vi "Op-Amp Test System.vi"() -> ()   [LabVIEW 2019]
uses:
  <vilib>/VirtualBench/VirtualBench.lvlib
  <vilib>/VirtualBench/_PS Configure Voltage Output0.vi
  <vilib>/VirtualBench/_MSO Configure Digital Edge Trigger0.vi
  <vilib>/VirtualBench/_MSO Configure Analog Edge Trigger0.vi
  <vilib>/VirtualBench/_MSO Configure Digital Pattern Trigger0.vi
  <vilib>/VirtualBench/_FGEN Configure Standard Waveform4.vi
  <vilib>/VirtualBench/_MSO Configure Timing12.vi
  <vilib>/Utility/error.llb/DialogType.ctl
  <vilib>/VirtualBench/_MSO Configure Analog Channel28.vi
  <vilib>/VirtualBench/_DMM Configure Measurement2.vi
  <vilib>/VirtualBench/_FGEN Configure Standard Waveform14.vi
  <vilib>/VirtualBench/_MSO Configure Analog Channel29.vi
  <vilib>/DigilentWF/DigilentWF.lvlib
panel:
  out "测试进度":u8(slide)=100 caption="Testing..." scale=0.0..100.0
  in  "开始测试":bool caption="Start"
  out "Slew Rate(V/us)":dbl format="%#.2f"
  out "Iin+(mA)":dbl format="%#.2g"
  out "Voffset(mV)":dbl=0.00017364742031570723 format="%#.2f"
  out "Iin-(mA)":dbl format="%#.2g"
  in  "图表选项卡":enum32{"Time Domain", "Frequency Domain"}(tab)=enum."Frequency Domain"
  out "Time Domain":waveform(dbl)(graph)={"t0"=timestamp(3648703829.272387 s since 1904-01-01), "dt"=5e-06, "Y"=[], "attributes"=variant("NI_ChannelName"=variant(string "mso/1"), "NI_UnitDescription"=variant(string "Volts"))}
  out "Amplitude-frequency":cluster{dbl[], dbl[]}(graph) caption="Amplitude-frequency characteristic"
  out "PSRR(dB)":dbl format="%#.1f"
  out "KCMRR(dB)":dbl format="%#.1f"
  out "Iin_mean(mA)":dbl format="%#.2g"
  out "Iin_bias(mA)":dbl format="%#.5g"
  out "K0(dB)":dbl format="%#.1f"
  in  "测试参数选项卡":T1(tab)=enum."Slew Rate"
  in  "Current PWS":T2={"PWS Channel"="VB8012-3126A15/ps/+25V", "Voltage Level (V)"=10.0, "Current Limit (A)"=0.05} {"Voltage Level (V)" min=0.0 max=12.0}
  in  "DC Offset(V)":dbl=1.0 caption="DC Offset" format="%#_13g"
  in  "Waveform Function":enum16{"Sine", "Square", "Triangle/Ramp", "DC"}(ring)=enum."DC"
  in  "CMRR PWS 2":T3={"PWS Channel 2"="VB8012-3126A15/ps/-25V", "Voltage Level (V)"=[-9.5, -8.5], "Current Limit (A)"=0.05} {"Voltage Level (V)" min=-12.0 max=0.0}
  in  "CMRR PWS1":T4={"PWS Channel 1"="VB8012-3126A15/ps/+25V", "Voltage Level (V)"=[9.5, 10.5], "Current Limit (A)"=0.05} {"Voltage Level (V)" min=0.0 max=12.0}
  in  "PSRR PWS":T5={"PWS Channel"="VB8012-3126A15/ps/+25V", "Voltage Level (V)"=[9.5, 10.0], "Current Limit (A)"=0.05} {"Voltage Level (V)" min=0.0 max=12.0}
  in  "Slew Rate PWS":T2={"PWS Channel"="VB8012-3126A15/ps/+25V", "Voltage Level (V)"=10.0, "Current Limit (A)"=0.05} {"Voltage Level (V)" min=0.0 max=12.0}
  in  "Frequency":dbl=20000.0 format="%#_13g"
  in  "Slewrate Waveform":enum16{"Sine", "Square", "Triangle/Ramp", "DC"}(ring)=enum."Square" caption="Waveform Function"
  in  "Amplitude":dbl=3.0 format="%#_13g"
  in  "DC Offset":dbl format="%#_13g"
  in  "Channel":tag="VB8012-3126A15/mso/1"
  in  "Vertical Range":dbl=3.0 format="%#_13g"
  in  "Trigger Type":T6(tab)
  in  "Digital Trigger Source":tag="mso/d0" caption="Trigger Source (no change)"
  in  "Edge":i32(ring) caption="Trigger Slope (no change)" items=["Rising", "Falling", "Either"]
  in  "Level (V)":dbl=0.4 format="%0.2f"
  in  "Hysteresis (V)":dbl=0.17
  in  "Analog Trigger Source":tag="VB8012-3126A15/mso/1" caption="Trigger Source (no change)"
  in  "Slope":i32(ring) caption="Trigger Slope (no change)" items=["Rising", "Falling", "Either"]
  in  "Pattern Trigger Source":tag="mso/d0:7" caption="Trigger Source (no change)"
  in  "Trigger Pattern":string="1R0XX1X0" caption="Trigger Pattern (no change)"
  in  "BW PWS":T2={"PWS Channel"="VB8012-3126A15/ps/+25V", "Voltage Level (V)"=10.0, "Current Limit (A)"=0.05} {"Voltage Level (V)" min=0.0 max=12.0}
  in  "Slewrate Waveform":enum16{"Sine", "Square", "Triangle/Ramp", "DC"}(ring) caption="Waveform Function"
  in  "Amplitude":dbl=2.0 format="%#_13g"
  in  "DC Offset":dbl format="%#_13g"
  in  "Vertical Range":dbl=3.0 format="%#_13g"
  in  "Channel":tag="VB8012-3126A15/mso/1"
  in  "Trigger Type":T6(tab)
  in  "Digital Trigger Source":tag="mso/d0" caption="Trigger Source (no change)"
  in  "Edge":i32(ring) caption="Trigger Slope (no change)" items=["Rising", "Falling", "Either"]
  in  "Analog Trigger Source":tag="mso/1" caption="Trigger Source (no change)"
  in  "Slope":i32(ring) caption="Trigger Slope (no change)" items=["Rising", "Falling", "Either"]
  in  "Level (V)":dbl format="%0.2f"
  in  "Hysteresis (V)":dbl=0.17
  in  "Pattern Trigger Source":tag="mso/d0:7" caption="Trigger Source (no change)"
  in  "Trigger Pattern":string="1R0XX1X0" caption="Trigger Pattern (no change)"
  in  "测试机台选择":tag="VB8012-3126A15"
  # "基于IECUBE-3839的运放自动化测试程序"
  # "硬件配置"
  # "DUT测试参数"
  # "设备选择"
  # "DUT测试结果"
  # "电源配置"
  # "函数发生器配置"
  # "电源配置"
  # "电源配置"
  # "电源配置"
  # "函数发生器配置"
  # "逻辑分析仪配置"
  # "Triggers immediately after MSO Run VI executes."
  # "电源配置"
  # "函数发生器配置"
  # "逻辑分析仪配置"
  # "Triggers immediately after MSO Run VI executes."
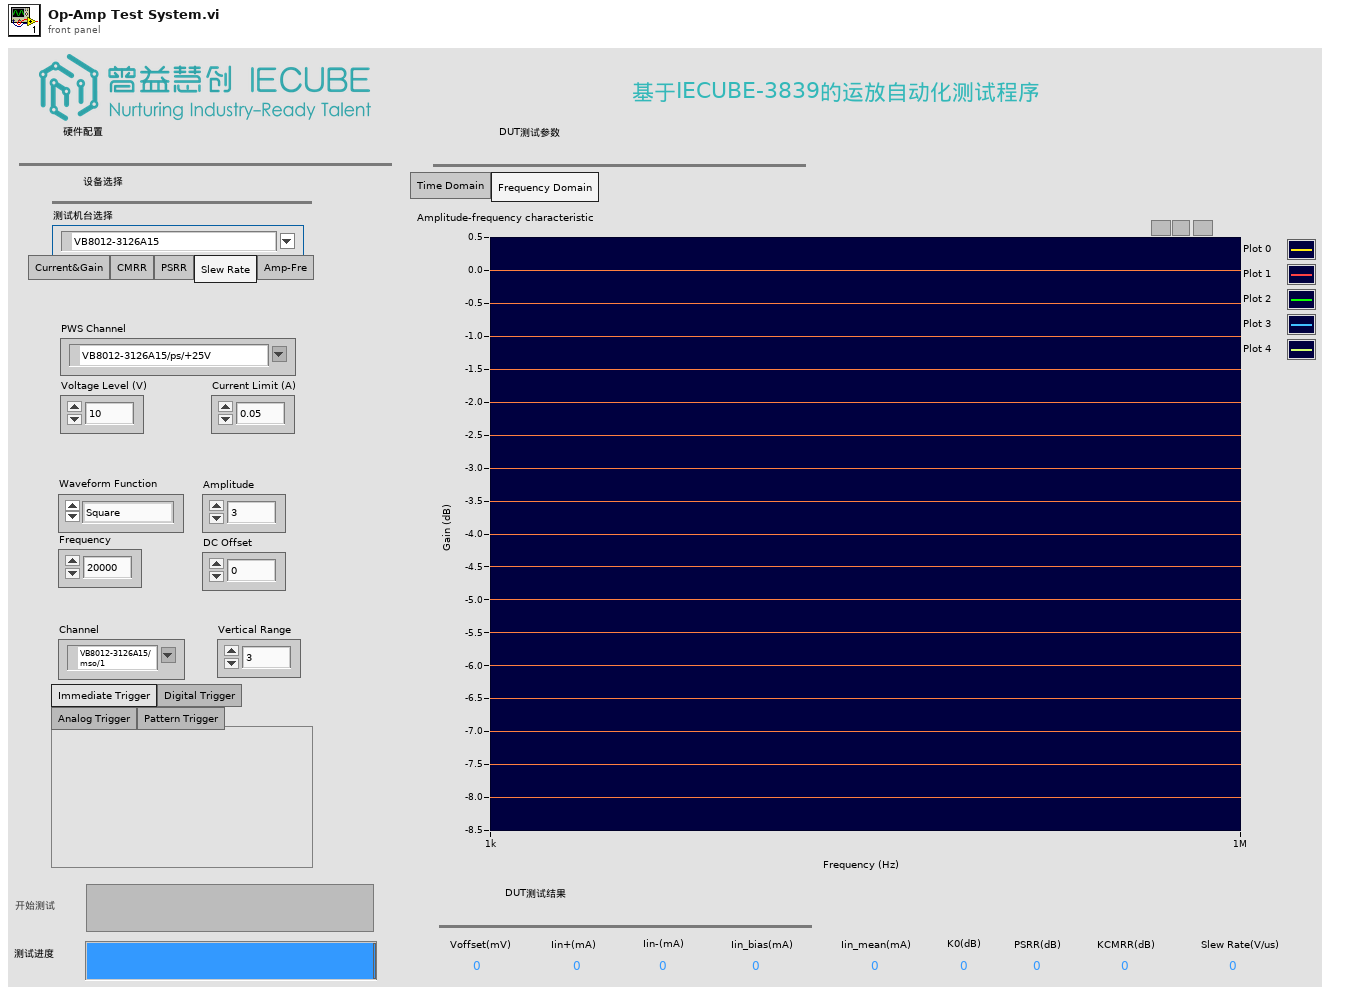
[diagram p1: front panel]
types:
  T1 = enum32{"Current&Gain", "CMRR", "PSRR", "Slew Rate", "Amp-Fre"}
  T2 = cluster{"PWS Channel":tag, "Voltage Level (V)":dbl, "Current Limit (A)":dbl}
  T3 = cluster{"PWS Channel 2":tag, "Voltage Level (V)":dbl[], "Current Limit (A)":dbl}
  T4 = cluster{"PWS Channel 1":tag, "Voltage Level (V)":dbl[], "Current Limit (A)":dbl}
  T5 = cluster{"PWS Channel":tag, "Voltage Level (V)":dbl[], "Current Limit (A)":dbl}
  T6 = enum32{"Immediate Trigger", "Digital Trigger", "Analog Trigger", "Pattern Trigger"}
  T7 = typedef "测试参数.ctl" = enum16{"Leakage Current", "Gain", "CMRR", "PSRR", "Slew Rate", "Amplitude-Frequency"}
  T8 = typedef "DialogType.ctl" = u16
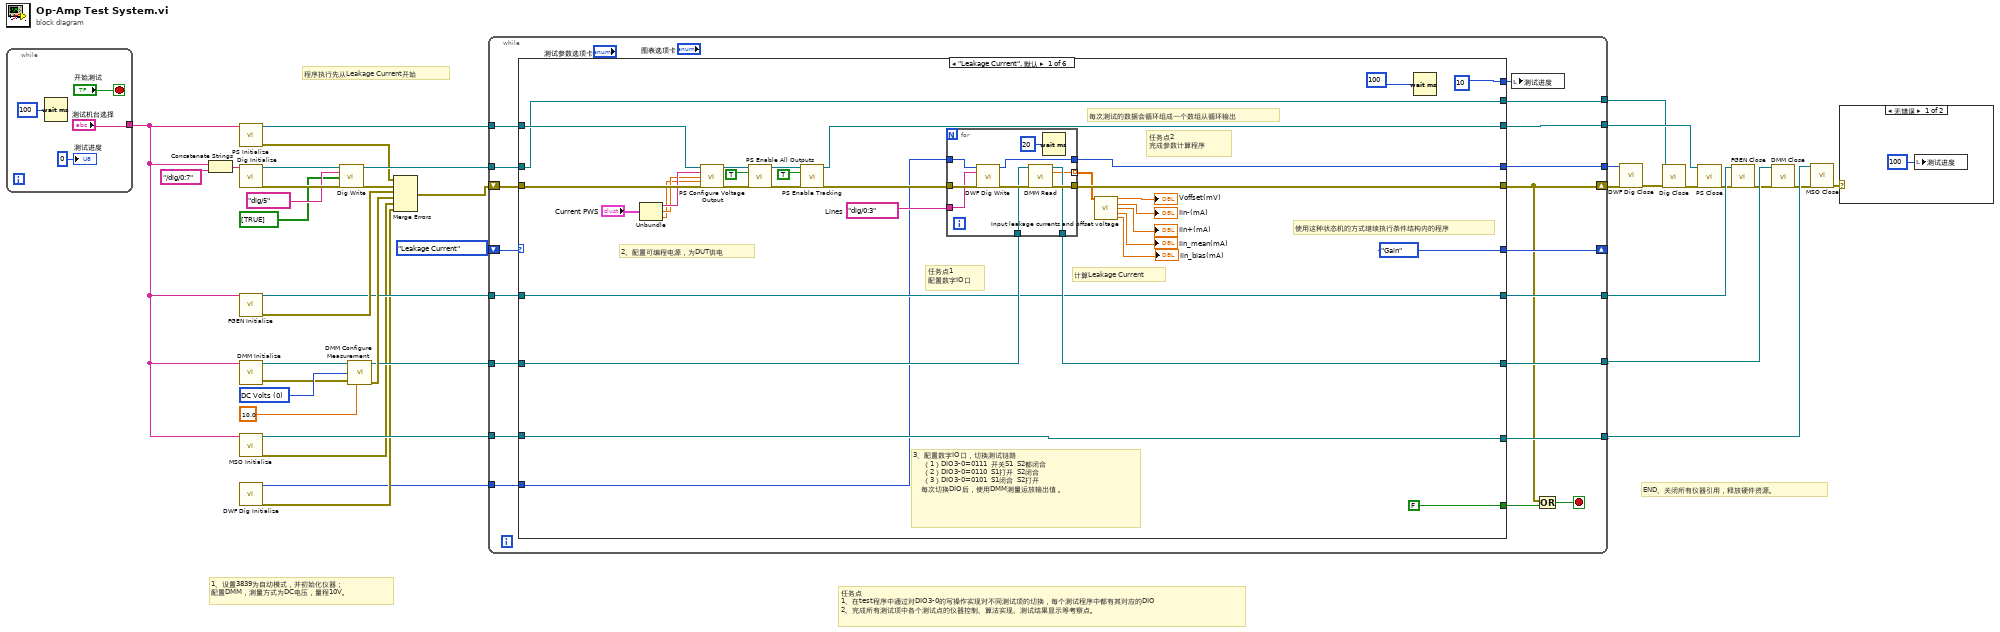
[diagram p0: block diagram]
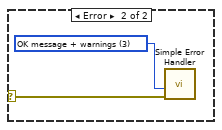
[diagram p2: hidden frame]
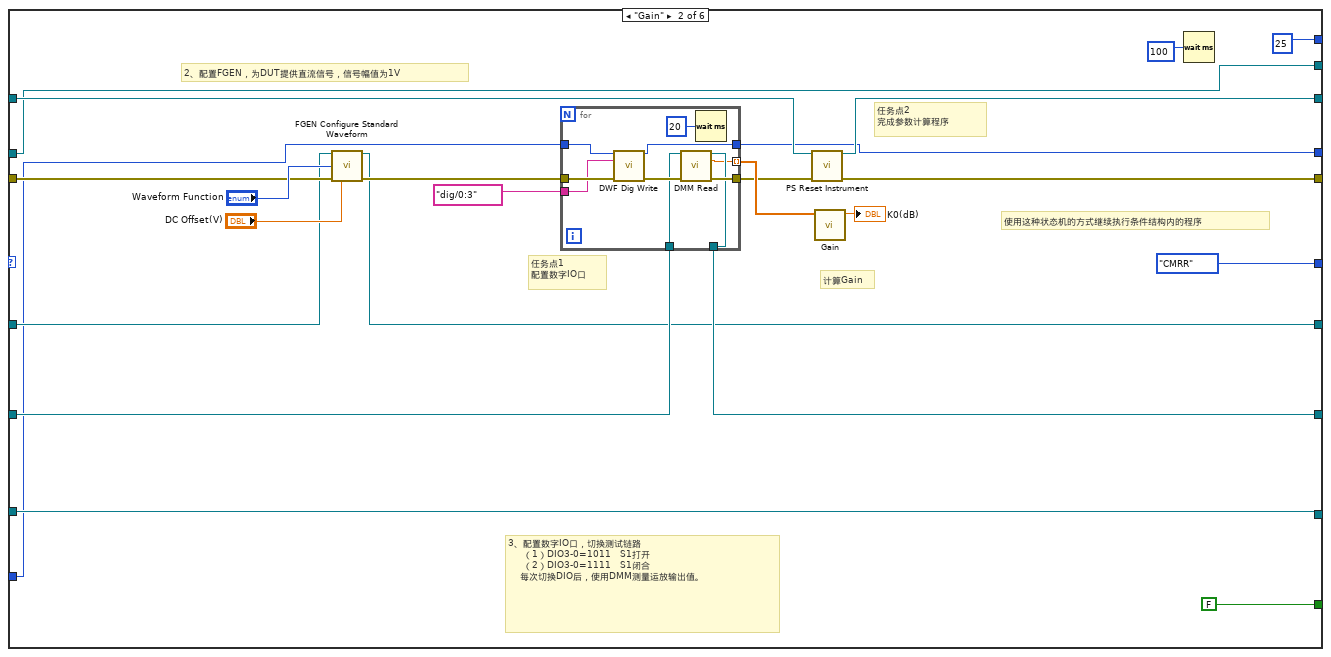
[diagram p3: hidden frame]
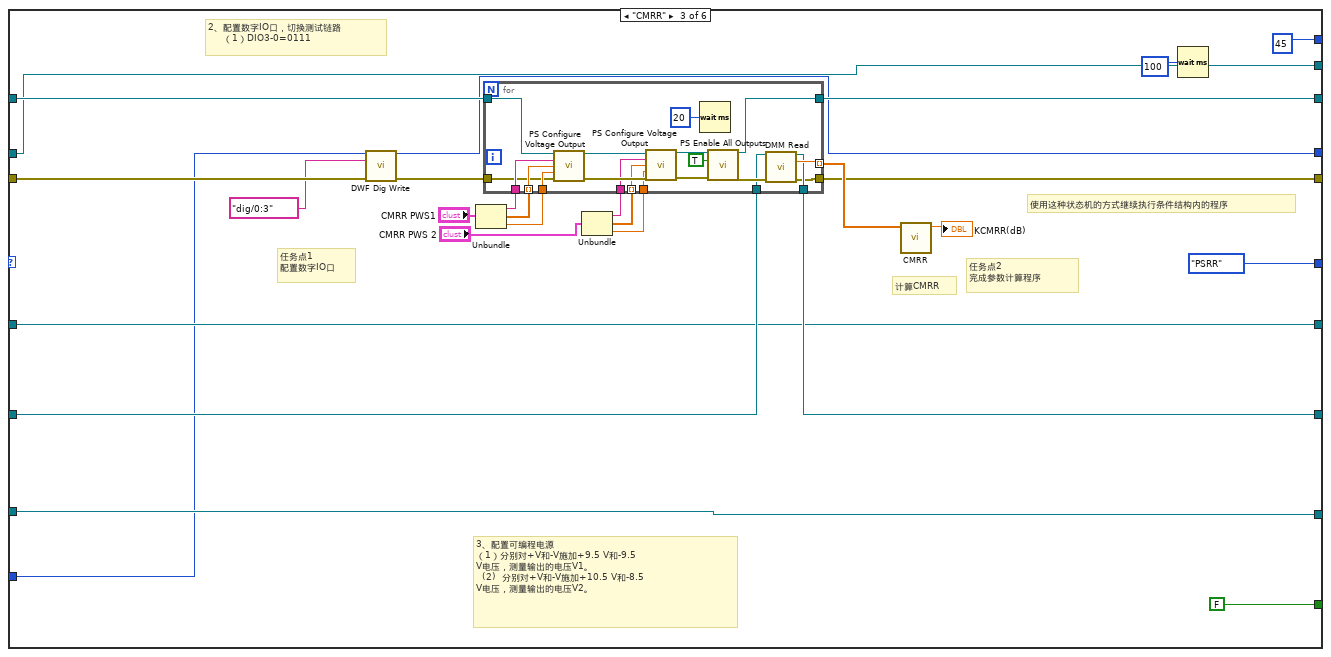
[diagram p4: hidden frame]
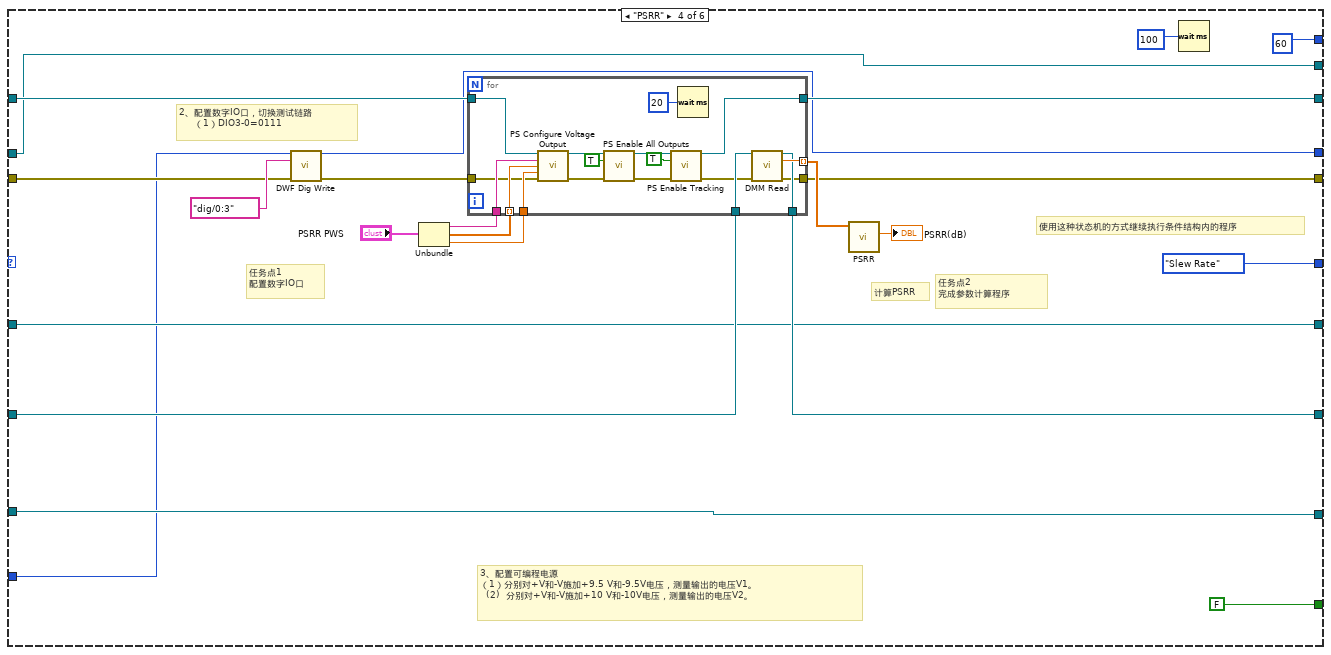
[diagram p5: hidden frame]
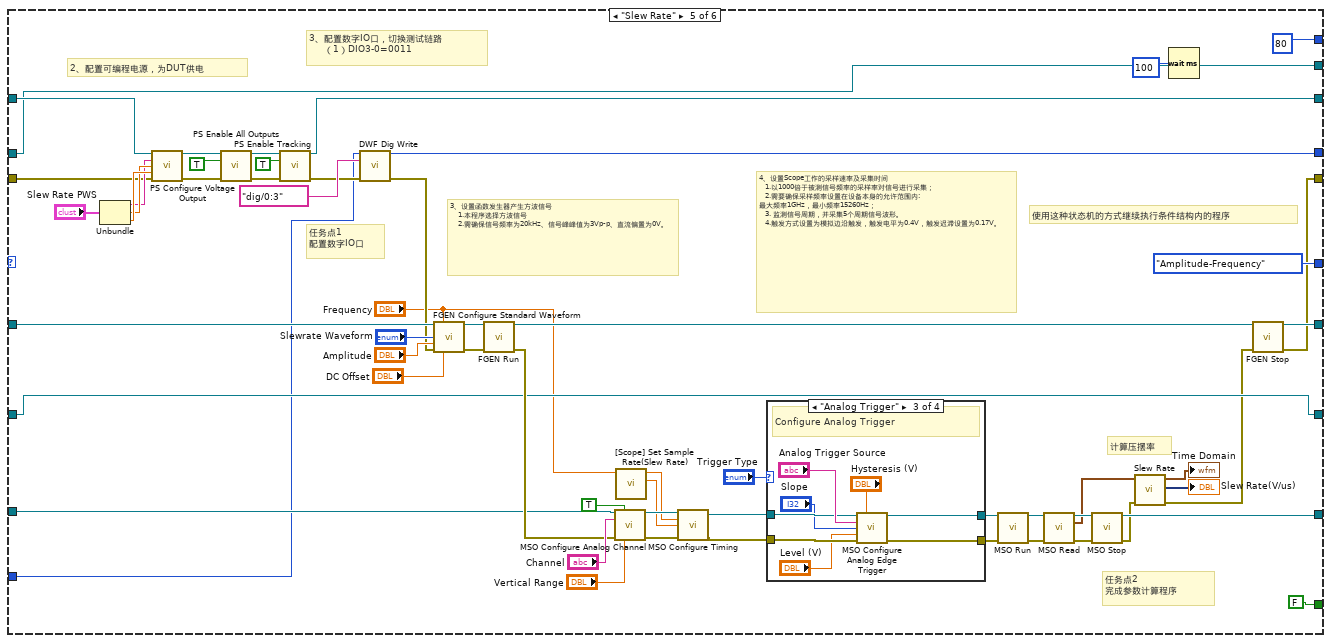
[diagram p6: hidden frame]
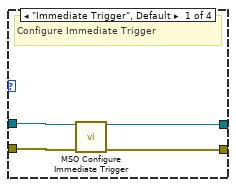
[diagram p7: hidden frame]
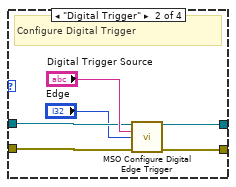
[diagram p8: hidden frame]
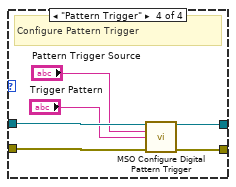
[diagram p9: hidden frame]
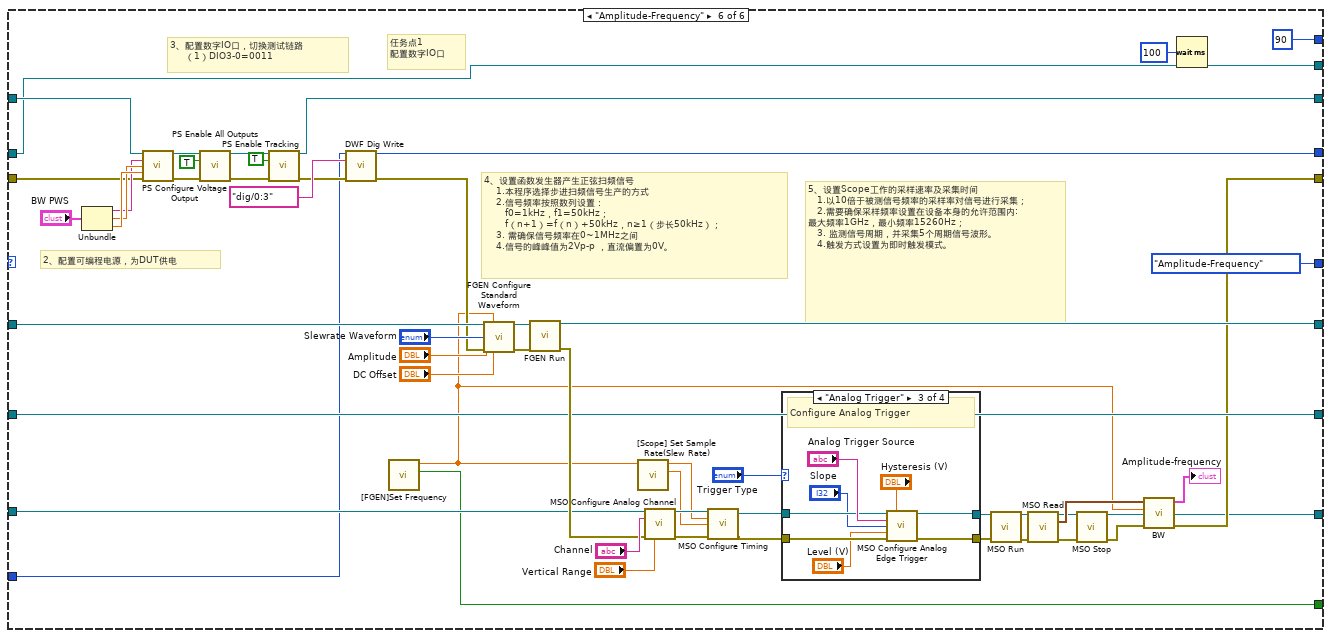
[diagram p10: hidden frame]
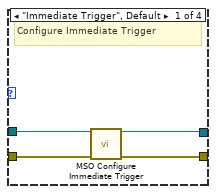
[diagram p11: hidden frame]
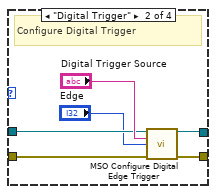
[diagram p12: hidden frame]
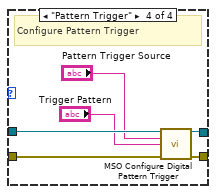
[diagram p13: hidden frame]
diagram:
  w28 = 0 items=["DC Volts", "AC Volts", "DC Current", "AC Current", "Resistance", "Diode"] ("Function")
  # "任务点\n1、在test程序中通过对DIO3-0的写操作实现对不同测试项的切换，每个测试程序中都有其对应的DIO\n2、完成所有测试项中各个测试点的仪器控制、算法实现、测试结果显示等考察点。"
  # "程序执行先从Leakage Current开始"
  # "END、关闭所有仪器引用，释放硬件资源。"
  # "1、设置3839为自动模式，并初始化仪器；\n配置DMM，测量方式为DC电压，量程10V。"
  n1 = while {
    tunnel: ["测试机台选择"] -> w15
    stop <- "开始测试" stop-if-true
    n2 = Wait (ms)(milliseconds to wait=u32 100 ("等待时间（毫秒）")) -> ()  [unwired: 1 out]
    "测试进度" <- u8 0 ("测试进度")
  }
  n3 = Concatenate Strings(w15, "/dig/0:7" ("字符串")) -> (w33:string)
  n4 = call <vilib>:"PS Initialize.vi"("Device Name"=w15) -> ("Instrument Handle Out"=w32:refnum<k21>, "Error Out"=w12:errorcluster)  [unwired: 13 in]
  n5 = call <vilib>:"Dig Initialize.vi"("Lines"=w33) -> ("Instrument Handle Out"=w38:refnum<k21>, "Error Out"=w37:errorcluster)  [unwired: 13 in]
  n6 = call <vilib>:"FGEN Initialize.vi"("Device Name"=w15) -> ("Instrument Handle Out"=w21:refnum<k21>, "Error Out"=w22:errorcluster)  [unwired: 13 in]
  n7 = call <vilib>:"DMM Initialize.vi"("Device Name"=w15) -> ("Instrument Handle Out"=w26:refnum<k21>, "Error Out"=w27:errorcluster)  [unwired: 13 in]
  n8 = call <vilib>:"MSO Initialize.vi"("Device Name"=w15) -> ("Instrument Handle Out"=w14:refnum<k21>, "Error Out"=w13:errorcluster)  [unwired: 13 in]
  n9 = call <vilib>:"DWF Dig Initialize.vi"() -> ("Instrument Handle Out"=w4:u32, "Error Out"=w5:errorcluster)  [unwired: 14 in]
  n10 = call <vilib>:"Dig Write.vi"("Instrument Handle In"=w38, "Lines"=tag "dig/5", "Data"=bool[] [TRUE], "Error In"=w37) -> ("Instrument Handle Out"=w31:refnum<k21>, "Error Out"=w11:errorcluster)  [unwired: 10 in]
  n11 = call-poly <vilib>:"DMM Configure Measurement.vi"("Instrument Handle In"=w26, "Function"=w28, "Error In"=w27, "Manual Range"=10.0) -> ("Instrument Handle Out"=w24:refnum<k21>, "Error Out"=w25:errorcluster)  [unwired: 10 in]
  n12 = Merge Errors(w12, w11, w22, w25, w13, w5) -> (w29:errorcluster)
  n13 = while {
    tunnel: w31 -> [w59]
    tunnel: w32 -> [w57]
    shift-right: [w58] -> _
    shift-left: 测试参数."Leakage Current" -> [w61]
    tunnel: w24 -> [w56]
    tunnel: [w55] -> w18
    shift-right: [w47] -> w3
    shift-left: w29 -> [w60]
    tunnel: [w54] -> w20
    tunnel: [w53] -> w19
    tunnel: w21 -> [w52]
    tunnel: [w51] -> w17
    tunnel: [w50] -> w16
    tunnel: w14 -> [w49]
    tunnel: w4 -> [w44]
    tunnel: [w43] -> w1
    stop <- w45 stop-if-true
    n14 = case shown="\"Leakage Current\", 默认" w61 {
      tunnel: w60 -> [w81 w119 w143 w188 w248 w328]
      tunnel: w59 -> [w64 w107 w140 w187 w228 w310]
      tunnel: [测试参数."Gain" 测试参数."CMRR" 测试参数."PSRR" 测试参数."Slew Rate" 测试参数."Amplitude-Frequency" 测试参数."Amplitude-Frequency"] -> w58
      tunnel: w57 -> [w79 w110 w161 w204 w247 w327]
      tunnel: w56 -> [w91 w121 w158 w201 w234 w345]
      tunnel: [w64 w107 w140 w187 w228 w310] -> w55
      tunnel: [w89 w111 w147 w193 w243 w324] -> w47
      tunnel: [w88 w120 w157 w200 w234 w345] -> w54
      tunnel: [w75 w109 w144 w192 w239 w325] -> w53
      tunnel: w52 -> [w74 w118 w156 w199 w265 w344]
      tunnel: [w74 w116 w156 w199 w244 w343] -> w51
      tunnel: [w73 w115 w155 w198 w262 w315] -> w50
      tunnel: w49 -> [w73 w115 w155 w198 w264 w342]
      tunnel: [FALSE FALSE FALSE FALSE FALSE w312] -> w46
      tunnel: [10 25 45 60 80 90] -> w48
      tunnel: w44 -> [w63 w105 w138 w186 w227 w309]
      tunnel: [w62 w106 w139 w185 w226 w308] -> w43
      frame "Leakage Current", Default {
        w90 = tag "dig/0:3"  # Lines
        # "任务点2\n完成参数计算程序"
        # "任务点1\n配置数字IO口"
        # "使用这种状态机的方式继续执行条件结构内的程序"
        # "计算Leakage Current"
        # "每次测试的数据会循环组成一个数组从循环输出"
        # "3、配置数字IO口，切换测试链路\n     （1）DIO3-0=0111  开关S1  S2都闭合\n     （2）DIO3-0=0110  S1打开  S2闭合 \n     （3）DIO3-0=0101  S1闭合  S2打开\n    每次切换DIO后，使用DMM测量运放输出值 。"
        # "2、配置可编程电源，为DUT供电"
        n15 = Unbundle("Current PWS") -> ("PWS Channel"=w78:tag, "Voltage Level (V)"=w77:dbl, "Current Limit (A)"=w76:dbl)
        n16 = call-poly <vilib>:"PS Configure Voltage Output.vi"("Instrument Handle In"=w79, "Channel"=w78, "Voltage Level"=w77, "Current Limit"=w76, "Error In"=w81) -> ("Instrument Handle Out"=w87:refnum<k21>, "Error Out"=w86:errorcluster)  [unwired: 9 in]
        n17 = call <vilib>:"PS Enable All Outputs.vi"("Instrument Handle In"=w87, "Enable Outputs"=TRUE, "Error In"=w86) -> ("Instrument Handle Out"=w84:refnum<k21>, "Error Out"=w83:errorcluster)  [unwired: 11 in]
        n18 = call <vilib>:"PS Enable Tracking.vi"("Instrument Handle In"=w84, "Enable Tracking"=TRUE, "Error In"=w83) -> ("Instrument Handle Out"=w75:refnum<k21>, "Error Out"=w80:errorcluster)  [unwired: 11 in]
        n19 = for {
          tunnel: w80 -> [w104]
          tunnel: [w103] -> w89
          tunnel: [w102] -> w88
          tunnel: [w101] -> w70 mode=indexing
          tunnel: w91 -> [w99]
          tunnel: w63 -> [w98]
          tunnel: [w97] -> w62
          tunnel: w90 -> [w96]
          n20 = call <vilib>:"DWF Dig Write.vi"("Instrument Handle In"=w98, "Lines"=w96, "Error In"=w104) -> ("Instrument Handle Out"=w97:u32, "Error Out"=w100:errorcluster)  [unwired: 11 in]
          n21 = call <vilib>:"DMM Read.vi"("Instrument Handle In"=w99, "Error In"=w100) -> ("Instrument Handle Out"=w102:refnum<k21>, "Measurement"=w101:dbl, "Error Out"=w103:errorcluster)  [unwired: 11 in]
          n22 = Wait (ms)(milliseconds to wait=u32 20 ("等待时间（毫秒）")) -> ()  [unwired: 1 out]
        }
        n23 = call "Input leakage currents and offset voltage.vi"("数组输入"=w70) -> ("Voffset"=→"Voffset(mV)":dbl, "Iin-"=→"Iin-(mA)":dbl, "Iin+"=→"Iin+(mA)":dbl, "Iin_mean"=→"Iin_mean(mA)":dbl, "Iin_bias"=→"Iin_bias(mA)":dbl)  [unwired: 10 in]
        n24 = Wait (ms)(milliseconds to wait=u32 100 ("等待时间（毫秒）")) -> ()  [unwired: 1 out]
      }
      frame "Gain" {
        # "任务点2\n完成参数计算程序"
        # "任务点1\n配置数字IO口"
        # "计算Gain"
        # "使用这种状态机的方式继续执行条件结构内的程序"
        # "2、配置FGEN，为DUT提供直流信号，信号幅值为1V"
        # "3、配置数字IO口，切换测试链路\n     （1）DIO3-0=1011   S1打开\n     （2）DIO3-0=1111   S1闭合\n    每次切换DIO后，使用DMM测量运放输出值。"
        n25 = call-poly <vilib>:"FGEN Configure Standard Waveform.vi"("Instrument Handle In"=w118, "Waveform Function"="Waveform Function", "Error In"=w119, "DC Offset"="DC Offset(V)") -> ("Instrument Handle Out"=w116:refnum<k21>, "Error Out"=w124:errorcluster)  [unwired: 10 in]
        n26 = for {
          tunnel: w124 -> [w137]
          tunnel: [w136] -> w112
          tunnel: [w135] -> w120
          tunnel: [w134] -> w127 mode=indexing
          tunnel: w121 -> [w132]
          tunnel: w105 -> [w131]
          tunnel: [w129] -> w106
          tunnel: tag "dig/0:3" ("Lines") -> [w128]
          n27 = call <vilib>:"DWF Dig Write.vi"("Instrument Handle In"=w131, "Lines"=w128, "Error In"=w137) -> ("Instrument Handle Out"=w129:u32, "Error Out"=w133:errorcluster)  [unwired: 11 in]
          n28 = call <vilib>:"DMM Read.vi"("Instrument Handle In"=w132, "Error In"=w133) -> ("Instrument Handle Out"=w135:refnum<k21>, "Measurement"=w134:dbl, "Error Out"=w136:errorcluster)  [unwired: 11 in]
          n29 = Wait (ms)(milliseconds to wait=u32 20 ("等待时间（毫秒）")) -> ()  [unwired: 1 out]
        }
        n30 = call <vilib>:"PS Reset Instrument.vi"("Instrument Handle In"=w110, "Error In"=w112) -> ("Instrument Handle Out"=w109:refnum<k21>, "Error Out"=w111:errorcluster)  [unwired: 12 in]
        n31 = call "Gain.vi"("数组"=w127) -> ("K0"=→"K0(dB)":dbl)  [unwired: 10 in]
        n32 = Wait (ms)(milliseconds to wait=u32 100 ("等待时间（毫秒）")) -> ()  [unwired: 1 out]
      }
      frame "CMRR" {
        # "任务点2\n完成参数计算程序"
        # "任务点1\n配置数字IO口"
        # "计算CMRR"
        # "使用这种状态机的方式继续执行条件结构内的程序"
        # "3、配置可编程电源\n（1）分别对+V和-V施加+9.5 V和-9.5 V电压，测量输出的电压V1。\n  (2)  分别对+V和-V施加+10.5 V和-8.5 V电压，测量输出的电压V2。"
        # "2、配置数字IO口，切换测试链路\n     （1）DIO3-0=0111"
        n33 = call <vilib>:"DWF Dig Write.vi"("Instrument Handle In"=w138, "Lines"=tag "dig/0:3", "Error In"=w143) -> ("Instrument Handle Out"=w139:u32, "Error Out"=w142:errorcluster)  [unwired: 11 in]
        n34 = Unbundle("CMRR PWS1") -> ("PWS Channel 1"=w162:tag, "Voltage Level (V)"=w163:dbl[], "Current Limit (A)"=w164:dbl)
        n35 = Unbundle("CMRR PWS 2") -> ("PWS Channel 2"=w150:tag, "Voltage Level (V)"=w149:dbl[], "Current Limit (A)"=w148:dbl)
        n36 = for {
          tunnel: w164 -> [w184]
          tunnel: w163 -> [w183] mode=indexing
          tunnel: w161 -> [w182]
          tunnel: w162 -> [w181]
          tunnel: w142 -> [w180]
          tunnel: w158 -> [w177]
          tunnel: [w176] -> w160 mode=indexing
          tunnel: [w175] -> w157
          tunnel: [w174] -> w147
          tunnel: w150 -> [w169]
          tunnel: w149 -> [w168] mode=indexing
          tunnel: w148 -> [w167]
          tunnel: [w166] -> w144
          n37 = call-poly <vilib>:"PS Configure Voltage Output.vi"("Instrument Handle In"=w182, "Channel"=w181, "Voltage Level"=w183, "Current Limit"=w184, "Error In"=w180) -> ("Instrument Handle Out"=w173:refnum<k21>, "Error Out"=w172:errorcluster)  [unwired: 9 in]
          n38 = call-poly <vilib>:"PS Configure Voltage Output.vi"("Instrument Handle In"=w173, "Channel"=w169, "Voltage Level"=w168, "Current Limit"=w167, "Error In"=w172) -> ("Instrument Handle Out"=w170:refnum<k21>, "Error Out"=w171:errorcluster)  [unwired: 9 in]
          n39 = Wait (ms)(milliseconds to wait=u32 20 ("等待时间（毫秒）")) -> ()  [unwired: 1 out]
          n40 = call <vilib>:"PS Enable All Outputs.vi"("Instrument Handle In"=w170, "Enable Outputs"=TRUE ("Enable Output"), "Error In"=w171) -> ("Instrument Handle Out"=w166:refnum<k21>, "Error Out"=w178:errorcluster)  [unwired: 11 in]
          n41 = call <vilib>:"DMM Read.vi"("Instrument Handle In"=w177, "Error In"=w178) -> ("Instrument Handle Out"=w175:refnum<k21>, "Measurement"=w176:dbl, "Error Out"=w174:errorcluster)  [unwired: 11 in]
        }
        n42 = call "CMRR.vi"("数组"=w160) -> ("KCMRR"=→"KCMRR(dB)":dbl)  [unwired: 10 in]
        n43 = Wait (ms)(milliseconds to wait=u32 100 ("等待时间（毫秒）")) -> ()  [unwired: 1 out]
      }
      frame "PSRR" {
        # "任务点2\n完成参数计算程序"
        # "任务点1\n配置数字IO口"
        # "使用这种状态机的方式继续执行条件结构内的程序"
        # "计算PSRR"
        # "3、配置可编程电源\n（1）分别对+V和-V施加+9.5 V和-9.5V电压，测量输出的电压V1。\n  (2)  分别对+V和-V施加+10 V和-10V电压，测量输出的电压V2。"
        # "2、配置数字IO口，切换测试链路\n     （1）DIO3-0=0111"
        n44 = call <vilib>:"DWF Dig Write.vi"("Instrument Handle In"=w186, "Lines"=tag "dig/0:3", "Error In"=w188) -> ("Instrument Handle Out"=w185:u32, "Error Out"=w189:errorcluster)  [unwired: 11 in]
        n45 = Unbundle("PSRR PWS") -> ("PWS Channel"=w205:tag, "Voltage Level (V)"=w206:dbl[], "Current Limit (A)"=w207:dbl)
        n46 = for {
          tunnel: w207 -> [w225]
          tunnel: w206 -> [w224] mode=indexing
          tunnel: w204 -> [w223]
          tunnel: w205 -> [w222]
          tunnel: w189 -> [w221]
          tunnel: w201 -> [w219]
          tunnel: [w218] -> w203 mode=indexing
          tunnel: [w217] -> w200
          tunnel: [w216] -> w193
          tunnel: [w211] -> w192
          n47 = call-poly <vilib>:"PS Configure Voltage Output.vi"("Instrument Handle In"=w223, "Channel"=w222, "Voltage Level"=w224, "Current Limit"=w225, "Error In"=w221) -> ("Instrument Handle Out"=w215:refnum<k21>, "Error Out"=w214:errorcluster)  [unwired: 9 in]
          n48 = call <vilib>:"PS Enable All Outputs.vi"("Instrument Handle In"=w215, "Enable Outputs"=TRUE ("Enable Output"), "Error In"=w214) -> ("Instrument Handle Out"=w212:refnum<k21>, "Error Out"=w213:errorcluster)  [unwired: 11 in]
          n49 = call <vilib>:"PS Enable Tracking.vi"("Instrument Handle In"=w212, "Enable Tracking"=TRUE, "Error In"=w213) -> ("Instrument Handle Out"=w211:refnum<k21>, "Error Out"=w210:errorcluster)  [unwired: 11 in]
          n50 = Wait (ms)(milliseconds to wait=u32 20 ("等待时间（毫秒）")) -> ()  [unwired: 1 out]
          n51 = call <vilib>:"DMM Read.vi"("Instrument Handle In"=w219, "Error In"=w210) -> ("Instrument Handle Out"=w217:refnum<k21>, "Measurement"=w218:dbl, "Error Out"=w216:errorcluster)  [unwired: 11 in]
        }
        n52 = call "PSRR.vi"("数组"=w203) -> ("PSRR"=→"PSRR(dB)":dbl)  [unwired: 10 in]
        n53 = Wait (ms)(milliseconds to wait=u32 100 ("等待时间（毫秒）")) -> ()  [unwired: 1 out]
      }
      frame "Slew Rate" {
        # "任务点2\n完成参数计算程序"
        # "任务点1\n配置数字IO口"
        # "计算压摆率"
        # "使用这种状态机的方式继续执行条件结构内的程序"
        # "3、配置数字IO口，切换测试链路\n     （1）DIO3-0=0011"
        # "4、设置Scope工作的采样速率及采集时间\n   1.以1000倍于被测信号频率的采样率对信号进行采集；\n   2.需要确保采样频率设置在设备本身的允许范围内: 最大频率1GHz，最小频率15260Hz；\n   3. 监测信号周期，并采集5个周期信号波形。\n   4.触发方式设置为模拟边沿触发，触发电平为0.4V，触发迟滞设置为0.17V。"
        # "3、设置函数发生器产生方波信号\n    1.本程序选择方波信号\n    2.需确保信号频率为20kHz、信号峰峰值为3Vp-p、直流偏置为0V。"
        # "2、配置可编程电源，为DUT供电"
        n54 = Unbundle("Slew Rate PWS") -> ("PWS Channel"=w253:tag, "Voltage Level (V)"=w254:dbl, "Current Limit (A)"=w255:dbl)
        n55 = call-poly <vilib>:"PS Configure Voltage Output.vi"("Instrument Handle In"=w247, "Channel"=w253, "Voltage Level"=w254, "Current Limit"=w255, "Error In"=w248) -> ("Instrument Handle Out"=w250:refnum<k21>, "Error Out"=w251:errorcluster)  [unwired: 9 in]
        n56 = call <vilib>:"PS Enable All Outputs.vi"("Instrument Handle In"=w250, "Enable Outputs"=TRUE, "Error In"=w251) -> ("Instrument Handle Out"=w240:refnum<k21>, "Error Out"=w252:errorcluster)  [unwired: 11 in]
        n57 = call <vilib>:"PS Enable Tracking.vi"("Instrument Handle In"=w240, "Enable Tracking"=TRUE, "Error In"=w252) -> ("Instrument Handle Out"=w239:refnum<k21>, "Error Out"=w241:errorcluster)  [unwired: 11 in]
        n58 = call <vilib>:"DWF Dig Write.vi"("Instrument Handle In"=w227, "Lines"=tag "dig/0:3", "Error In"=w241) -> ("Instrument Handle Out"=w226:u32, "Error Out"=w256:errorcluster)  [unwired: 11 in]
        n59 = call-poly <vilib>:"FGEN Configure Standard Waveform.vi"("Instrument Handle In"=w265, "Frequency"="Frequency", "Waveform Function"="Slewrate Waveform", "Amplitude"="Amplitude", "Error In"=w256, "DC Offset"="DC Offset") -> ("Instrument Handle Out"=w279:refnum<k21>, "Error Out"=w280:errorcluster)  [unwired: 8 in]
        n60 = call <vilib>:"FGEN Run.vi"("Instrument Handle In"=w279, "Error In"=w280) -> ("Instrument Handle Out"=w245:refnum<k21>, "Error Out"=w275:errorcluster)  [unwired: 12 in]
        n61 = call-poly <vilib>:"MSO Configure Analog Channel.vi"("Instrument Handle In"=w264, "Enable Channel"=TRUE, "Channel"="Channel", "Error In"=w275, "Vertical Range"="Vertical Range") -> ("Instrument Handle Out"=w272:refnum<k21>, "Error Out"=w273:errorcluster)  [unwired: 9 in]
        n62 = call "[Scope] Set Sample Rate(Slew Rate).vi"("Frequency"="Frequency") -> ("Acquistion Time"=w229:dbl, "Sample Rate"=w230:dbl)  [unwired: 9 in]
        n63 = call-poly <vilib>:"MSO Configure Timing.vi"("Instrument Handle In"=w272, "Sample Rate"=w230, "Acquisition Time (s)"=w229, "Error In"=w273) -> ("Instrument Handle Out"=w271:refnum<k21>, "Error Out"=w270:errorcluster)  [unwired: 10 in]
        n64 = case shown="\"Analog Trigger\"" "Trigger Type" {
          tunnel: w271 -> [w287 w290 w295 w305]
          tunnel: w270 -> [w285 w292 w300 w303]
          tunnel: [w286 w289 w296 w306] -> w268
          tunnel: [w284 w293 w299 w307] -> w269
          frame "Immediate Trigger", Default {
            # "Configure Immediate Trigger"
            n65 = call <vilib>:"MSO Configure Immediate Trigger.vi"("Instrument Handle In"=w287, "Error In"=w285) -> ("Instrument Handle Out"=w286:refnum<k21>, "Error Out"=w284:errorcluster)  [unwired: 12 in]
          }
          frame "Digital Trigger" {
            # "Configure Digital Trigger"
            n66 = call-poly <vilib>:"MSO Configure Digital Edge Trigger.vi"("Instrument Handle In"=w290, "Trigger Source"="Digital Trigger Source", "Trigger Slope"="Edge", "Error In"=w292) -> ("Instrument Handle Out"=w289:refnum<k21>, "Error Out"=w293:errorcluster)  [unwired: 10 in]
          }
          frame "Analog Trigger" {
            # "Configure Analog Trigger"
            n67 = call-poly <vilib>:"MSO Configure Analog Edge Trigger.vi"("Instrument Handle In"=w295, "Trigger Hysteresis"="Hysteresis (V)", "Trigger Source"="Analog Trigger Source", "Trigger Slope"="Slope", "Trigger Level"="Level (V)", "Error In"=w300) -> ("Instrument Handle Out"=w296:refnum<k21>, "Error Out"=w299:errorcluster)  [unwired: 8 in]
          }
          frame "Pattern Trigger" {
            # "Configure Pattern Trigger"
            n68 = call-poly <vilib>:"MSO Configure Digital Pattern Trigger.vi"("Instrument Handle In"=w305, "Trigger Source"="Pattern Trigger Source", "Trigger Pattern"="Trigger Pattern", "Error In"=w303) -> ("Instrument Handle Out"=w306:refnum<k21>, "Error Out"=w307:errorcluster)  [unwired: 10 in]
          }
        }
        n69 = call <vilib>:"MSO Run.vi"("Instrument Handle In"=w268, "Error In"=w269) -> ("Instrument Handle Out"=w260:refnum<k21>, "Error Out"=w259:errorcluster)  [unwired: 12 in]
        n70 = call <vilib>:"MSO Read.vi"("Instrument Handle In"=w260, "Error In"=w259) -> ("Instrument Handle Out"=w266:refnum<k21>, "Analog Waveforms"=w258:waveform(dbl)[], "Error Out"=w261:errorcluster)  [unwired: 8 in, 3 out]
        n71 = call <vilib>:"MSO Stop.vi"("Instrument Handle In"=w266, "Error In"=w261) -> ("Instrument Handle Out"=w262:refnum<k21>, "Error Out"=w233:errorcluster)  [unwired: 12 in]
        n72 = call "Slew Rate.vi"("错误输入（无错误）"=w233, "Analog Waveforms"=w258) -> ("错误输出"=w232:errorcluster, "Dynamic Data"=→"Slew Rate(V/us)":dynamicdata, "waveform"=→"Time Domain":waveform(dbl))  [unwired: 7 in]
        n73 = Wait (ms)(milliseconds to wait=u32 100 ("等待时间（毫秒）")) -> ()  [unwired: 1 out]
        n74 = call <vilib>:"FGEN Stop.vi"("Instrument Handle In"=w245, "Error In"=w232) -> ("Instrument Handle Out"=w244:refnum<k21>, "Error Out"=w243:errorcluster)  [unwired: 12 in]
      }
      frame "Amplitude-Frequency" {
        # "任务点1\n配置数字IO口"
        # "3、配置数字IO口，切换测试链路\n     （1）DIO3-0=0011"
        # "5、设置Scope工作的采样速率及采集时间\n   1.以10倍于被测信号频率的采样率对信号进行采集；\n   2.需要确保采样频率设置在设备本身的允许范围内: 最大频率1GHz，最小频率15260Hz；\n   3. 监测信号周期，并采集5个周期信号波形。\n   4.触发方式设置为即时触发模式。"
        # "4、设置函数发生器产生正弦扫频信号\n    1.本程序选择步进扫频信号生产的方式\n    2.信号频率按照数列设置：\n       f0=1kHz，f1=50kHz；\n       f（n+1）=f（n）+50kHz，n≥1（步长50kHz）；\n    3. 需确保信号频率在0~1MHz之间\n    4.信号的峰峰值为2Vp-p ，直流偏置为0V。"
        # "2、配置可编程电源，为DUT供电"
        n75 = Unbundle("BW PWS") -> ("PWS Channel"=w335:tag, "Voltage Level (V)"=w336:dbl, "Current Limit (A)"=w337:dbl)
        n76 = call-poly <vilib>:"PS Configure Voltage Output.vi"("Instrument Handle In"=w327, "Channel"=w335, "Voltage Level"=w336, "Current Limit"=w337, "Error In"=w328) -> ("Instrument Handle Out"=w331:refnum<k21>, "Error Out"=w332:errorcluster)  [unwired: 9 in]
        n77 = call <vilib>:"PS Enable All Outputs.vi"("Instrument Handle In"=w331, "Enable Outputs"=TRUE, "Error In"=w332) -> ("Instrument Handle Out"=w333:refnum<k21>, "Error Out"=w334:errorcluster)  [unwired: 11 in]
        n78 = call <vilib>:"PS Enable Tracking.vi"("Instrument Handle In"=w333, "Enable Tracking"=TRUE, "Error In"=w334) -> ("Instrument Handle Out"=w325:refnum<k21>, "Error Out"=w326:errorcluster)  [unwired: 11 in]
        n79 = call <vilib>:"DWF Dig Write.vi"("Instrument Handle In"=w309, "Lines"=tag "dig/0:3", "Error In"=w326) -> ("Instrument Handle Out"=w308:u32, "Error Out"=w338:errorcluster)  [unwired: 11 in]
        n80 = call "[FGEN]Set Frequency.vi"() -> ("Freq in range?"=w312:bool, "Frequency"=w311:dbl)  [unwired: 10 in]
        n81 = call-poly <vilib>:"FGEN Configure Standard Waveform.vi"("Instrument Handle In"=w344, "Frequency"=w311, "Waveform Function"="Slewrate Waveform", "Amplitude"="Amplitude", "Error In"=w338, "DC Offset"="DC Offset") -> ("Instrument Handle Out"=w357:refnum<k21>, "Error Out"=w358:errorcluster)  [unwired: 8 in]
        n82 = call <vilib>:"FGEN Run.vi"("Instrument Handle In"=w357, "Error In"=w358) -> ("Instrument Handle Out"=w343:refnum<k21>, "Error Out"=w354:errorcluster)  [unwired: 12 in]
        n83 = call "[Scope] Set Sample Rate(Slew Rate).vi"("Frequency"=w311) -> ("Acquistion Time"=w313:dbl, "Sample Rate"=w314:dbl)  [unwired: 9 in]
        n84 = call-poly <vilib>:"MSO Configure Analog Channel.vi"("Instrument Handle In"=w342, "Channel"="Channel", "Error In"=w354, "Vertical Range"="Vertical Range") -> ("Instrument Handle Out"=w351:refnum<k21>, "Error Out"=w352:errorcluster)  [unwired: 10 in]
        n85 = call-poly <vilib>:"MSO Configure Timing.vi"("Instrument Handle In"=w351, "Sample Rate"=w314, "Acquisition Time (s)"=w313, "Error In"=w352) -> ("Instrument Handle Out"=w350:refnum<k21>, "Error Out"=w349:errorcluster)  [unwired: 10 in]
        n86 = case shown="\"Analog Trigger\"" "Trigger Type" {
          tunnel: w350 -> [w365 w368 w373 w383]
          tunnel: w349 -> [w363 w370 w378 w381]
          tunnel: [w364 w367 w374 w384] -> w347
          tunnel: [w362 w371 w377 w385] -> w348
          frame "Immediate Trigger", Default {
            # "Configure Immediate Trigger"
            n87 = call <vilib>:"MSO Configure Immediate Trigger.vi"("Instrument Handle In"=w365, "Error In"=w363) -> ("Instrument Handle Out"=w364:refnum<k21>, "Error Out"=w362:errorcluster)  [unwired: 12 in]
          }
          frame "Digital Trigger" {
            # "Configure Digital Trigger"
            n88 = call-poly <vilib>:"MSO Configure Digital Edge Trigger.vi"("Instrument Handle In"=w368, "Trigger Source"="Digital Trigger Source", "Trigger Slope"="Edge", "Error In"=w370) -> ("Instrument Handle Out"=w367:refnum<k21>, "Error Out"=w371:errorcluster)  [unwired: 10 in]
          }
          frame "Analog Trigger" {
            # "Configure Analog Trigger"
            n89 = call-poly <vilib>:"MSO Configure Analog Edge Trigger.vi"("Instrument Handle In"=w373, "Trigger Hysteresis"="Hysteresis (V)", "Trigger Source"="Analog Trigger Source", "Trigger Slope"="Slope", "Trigger Level"="Level (V)", "Error In"=w378) -> ("Instrument Handle Out"=w374:refnum<k21>, "Error Out"=w377:errorcluster)  [unwired: 8 in]
          }
          frame "Pattern Trigger" {
            # "Configure Pattern Trigger"
            n90 = call-poly <vilib>:"MSO Configure Digital Pattern Trigger.vi"("Instrument Handle In"=w383, "Trigger Source"="Pattern Trigger Source", "Trigger Pattern"="Trigger Pattern", "Error In"=w381) -> ("Instrument Handle Out"=w384:refnum<k21>, "Error Out"=w385:errorcluster)  [unwired: 10 in]
          }
        }
        n91 = call <vilib>:"MSO Run.vi"("Instrument Handle In"=w347, "Error In"=w348) -> ("Instrument Handle Out"=w341:refnum<k21>, "Error Out"=w340:errorcluster)  [unwired: 12 in]
        n92 = call <vilib>:"MSO Read.vi"("Instrument Handle In"=w341, "Error In"=w340) -> ("Instrument Handle Out"=w316:refnum<k21>, "Analog Waveforms"=w322:waveform(dbl)[], "Error Out"=w321:errorcluster)  [unwired: 8 in, 3 out]
        n93 = call <vilib>:"MSO Stop.vi"("Instrument Handle In"=w316, "Error In"=w321) -> ("Instrument Handle Out"=w315:refnum<k21>, "Error Out"=w317:errorcluster)  [unwired: 12 in]
        n94 = call "BW.vi"("错误输入（无错误）"=w317, "frequency"=w311, "Analog Waveforms"=w322) -> ("错误输出"=w324:errorcluster, "Gain Display"=→"Amplitude-frequency":cluster{dbl[], dbl[]})  [unwired: 7 in]
        n95 = Wait (ms)(milliseconds to wait=u32 100 ("等待时间（毫秒）")) -> ()  [unwired: 1 out]
      }
    }
    n96 = local write "测试进度"(w48) -> ()
    n97 = Or(x=w47, y=w46) -> (x .or. y?=w45:bool)
  }
  n98 = call <vilib>:"DWF Dig Close.vi"("Instrument Handle In"=w1, "Error In"=w3) -> ("Error Out"=w2:errorcluster)  [unwired: 13 in]
  n99 = call <vilib>:"Dig Close.vi"("Instrument Handle In"=w18, "Error In"=w2) -> ("Error Out"=w10:errorcluster)  [unwired: 13 in]
  n100 = call <vilib>:"PS Close.vi"("Instrument Handle In"=w19, "Error In"=w10) -> ("Error Out"=w9:errorcluster)  [unwired: 13 in]
  n101 = call <vilib>:"FGEN Close.vi"("Instrument Handle In"=w17, "Error In"=w9) -> ("Error Out"=w8:errorcluster)  [unwired: 13 in]
  n102 = call <vilib>:"DMM Close.vi"("Instrument Handle In"=w20, "Error In"=w8) -> ("Error Out"=w7:errorcluster)  [unwired: 13 in]
  n103 = call <vilib>:"MSO Close.vi"("Instrument Handle In"=w16, "Error In"=w7) -> ("Error Out"=w6:errorcluster)  [unwired: 13 in]
  n104 = case shown="无错误" w6 {
    selector: w6 -> [_ w387]
    frame No Error {
      n105 = local write "测试进度"(u8 100 ("测试进度")) -> ()
    }
    frame Error {
      w388 = T8 3 items=["no dialog", "OK message", "continue or stop message", "OK message + warnings", "continue/stop + warnings"] ("type of dialog (OK msg:1)")
      n106 = call <vilib>:"Simple Error Handler.vi"("type of dialog (OK msg:1)"=w388, "error in (no error)"=w387) -> ()  [unwired: 3 in, 5 out]
    }
  }
